vi "ProdaNG.Error.DefinedCodes.vi"() -> (5 "Defined codes out":i32[](array[numeric])=[0, 234], 6 "Error codes out":i32[](array[numeric])=[232, 12560, -12154, -1017], 7 "Descripotions out":string[](array[string])=["232: ERROR_NO_DATA system cannot be identified definely, check \n - system name is correct in TB.ini  or in DataBase,\n - single/double fixture indicator, \n - WabcoId", "ORA-12560: cannot open wrapper or prodllng.dll ", "ORA-12154:\tTNS:could not resolve the connect identifier specified\nCause:\tA connection to a database or other service was requested using a connect identifier, and the connect identifier specified could not be resolved into a connect descriptor using one of the naming methods configured. For example, if the type of connect identifier used was a net service name then the net service name could not be found in a naming method repository, or the repository could not be located or reached.", "ORA-1017 invalid username/password when trying to login as internal"])   [LabVIEW 2016]
doc: "OUTPUTS:\nDefined codes - codes which should not be treated as errors\n\nError codes - error codes from wrapper or dll\n\nDescriptions - descriptions of error codes from wrapper or dll"
panel:
  in  "Descripotions":string[](array[string])=["232: ERROR_NO_DATA system cannot be identified definely, check \n - system name is correct in TB.ini  or in DataBase,\n - single/double fixture indicator, \n - WabcoId", "12560: cannot open wrapper or prodllng.dll ", "ORA-12154:\tTNS:could not resolve the connect identifier specified\nCause:\tA connection to a database or other service was requested using a connect identifier, and the connect identifier specified could not be resolved into a connect descriptor using one of the naming methods configured. For example, if the type of connect identifier used was a net service name then the net service name could not be found in a naming method repository, or the repository could not be located or reached.", "ORA-1017 invalid username/password when trying to login as internal", "ORA-28000:\tthe account is locked\nCause:\tThe user has entered wrong password consequently for maximum number of times specified by the user's profile parameter FAILED_LOGIN_ATTEMPTS, or the DBA has locked the account", "ORA-2112: error when trying to store duplicated uniq no for products (two or more records with the same Wabco_Part_Id and Serial_Number in Product Table: select * from prodang.product a, prodang.product b where A.WABCO_PART_ID=B.WABCO_PART_ID and A.SERIAL_NUMBER=B.SERIAL_NUMBER and a.id<>b.id)\n\nORA-02112:\tPCC: SELECT..INTO returns too many rows\nCause:\tA SELECT...INTO statement returned more rows than can be stored in the host variable provided.\nAction:\tThere are three possible solutions:\n\n   1. Use the precompiler option SELECT_ERROR=NO.\n   2. Declare a host variable with a larger array dimension.\n   3. Declare a cursor or cursor variable for the select statement."]
  in  "Error codes":i32[](array[numeric])=[232, 12560, -12154, -1017, -28000, -2112]
  in  "Defined codes":i32[](array[numeric])=[0, 234]
  # "Description of codes:\n0: no error\n234: prodllng.dll info"
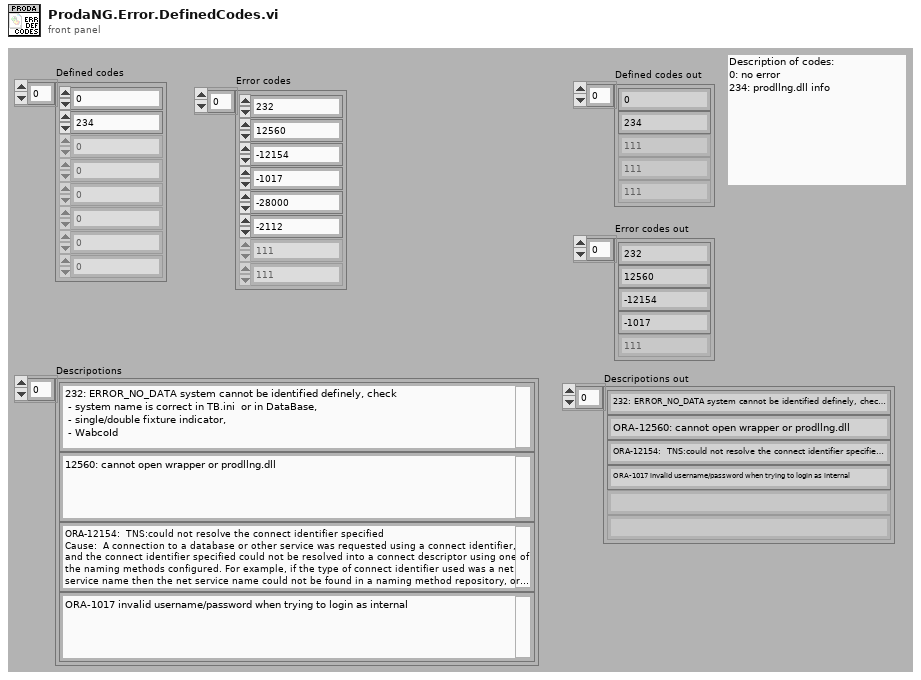
[diagram p1: front panel]
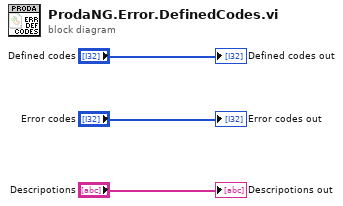
[diagram p0: block diagram]
diagram:
  "Defined codes out" <- "Defined codes"
  "Error codes out" <- "Error codes"
  "Descripotions out" <- "Descripotions"
